vi "AI-Freq1.vi"(7 "DAQConfigRef":T1, 8 "error in":errorcluster, 10 "Mode":string, 11 "CH":string) -> (0 "error out":errorcluster, 3 "波形图":waveform(dbl)(graph))   [LabVIEW 2013]
uses:
  Controls/DAQConfigRef.ctl
  Controls/DAQConfig.ctl
  <vilib>/DAQmx/read.llb/DAQmx Read (Analog Wfm 1Chan NSamp).vi
  <vilib>/DAQmx/create/channels.llb/DAQmx Create Channel (AI-Voltage-Basic).vi
  <vilib>/DAQmx/configure/timing.llb/DAQmx Timing (Sample Clock).vi
  <vilib>/DAQmx/miscellaneous.llb/DAQmx Fill In Error Info.vi
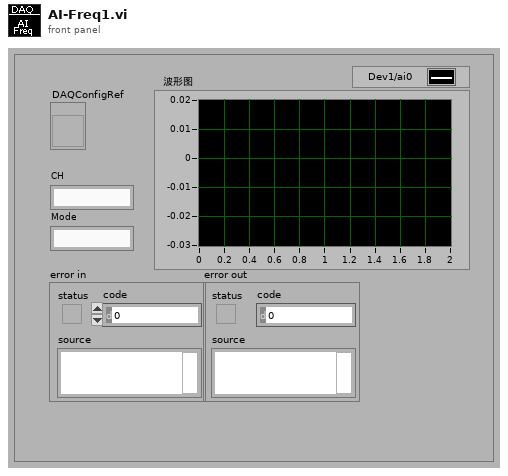
[diagram p1: front panel]
types:
  T1 = typedef "DAQConfigRef.ctl" = refnum<vi>
  T2 = typedef "DAQConfig.ctl" = cluster{"DIO":string[][], "AO":string[][], "AI":string[][]}
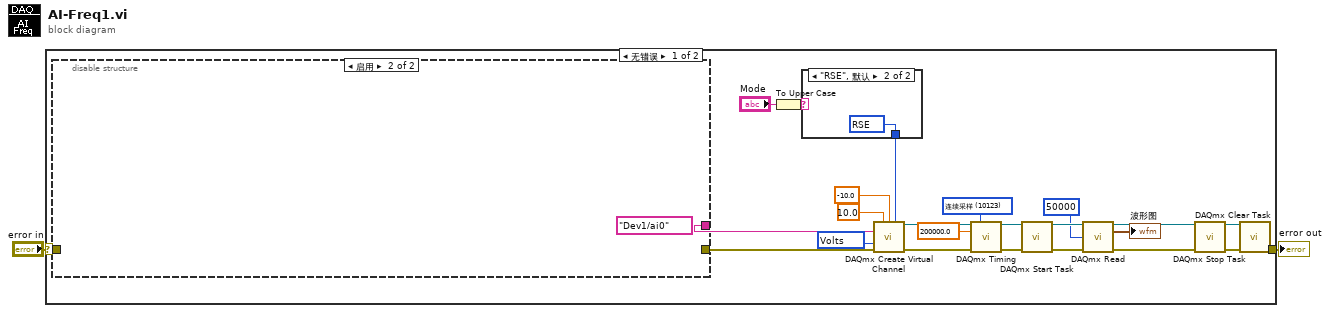
[diagram p0: block diagram]
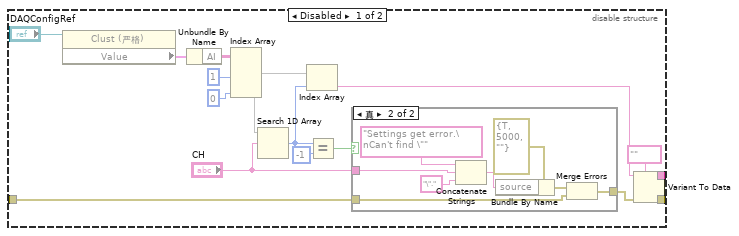
[diagram p2: hidden frame]
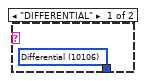
[diagram p4: hidden frame]
diagram:
  n1 = case shown="无错误" "error in" {
    selector: "error in" -> [w15 w56]
    tunnel: [w26 w56] -> w2
    frame No Error {
      w11 = 10123 items=["有限采样"=10178, "连续采样"=10123, "硬件定时单点"=12522] ("sample mode")
      w21 = 10348 items=["Volts"=10348, "From Custom Scale"=10065] ("units")
      n2 = disable-structure shown="启用" {
        disable-tunnel: [w31 tag "Dev1/ai0" ("lines")] -> w17
        disable-tunnel: [w30 _] -> w16
        disable-tunnel: w15 -> [w28 _]
        frame Disabled {
          n3 = property class="Clust (严格)"(reference="DAQConfigRef") -> ("Value"=w38:T2)  [unwired: 1 in, 2 out]
          n4 = Unbundle By Name(w38) -> ("AI"=w43:string[][])
          n5 = Index Array(array=w43, index (col) #1=1 ("索引 (行)"), index (col) #2=0 ("索引 (列)")) -> (element #1=w37:string[], element #2=w36:string[])  [unwired: 2 in]
          n6 = Search 1D Array(1D array=w36, element="CH") -> (index of element=w40:i32)  [unwired: 1 in]
          n7 = Index Array(array=w37, index=w40) -> (element=w27:string)
          n8 = Equal?(x=w40, y=-1) -> (x = y?=w34:bool)
          n9 = case shown="真" w34 {
            tunnel: w28 -> [w44 w47]
            tunnel: [w44 w46] -> w29
            tunnel: "CH" -> [_ w45]
            frame False {
            }
            frame True {
              n10 = Concatenate Strings("Settings get error.\nCan't find \"" ("message"), w45, "\"." ("string")) -> (w51:string)
              n11 = Bundle By Name(cluster=errorcluster {"status"=TRUE, "code"=5000, "source"=""} ("error in 1 (no error)"), "source"=w51) -> (w50:errorcluster)
              n12 = Merge Errors(w50, w47) -> (w46:errorcluster)
            }
          }
          n13 = Variant To Data(error in=w29, type=tag "" ("lines"), Variant=w27) -> (data=w31:tag, error out=w30:errorcluster)
        }
        frame Enabled {
        }
      }
      n14 = To Upper Case(1:"Mode") -> (0:w13:string)
      n15 = case shown="\"RSE\", 默认" w13 {
        tunnel: [w54 w55] -> w12
        frame "DIFFERENTIAL" {
          w54 = 10106 items=["default"=-1, "RSE"=10083, "NRSE"=10078, "Differential"=10106, "Pseudodifferential"=12529] ("input terminal configuration")
        }
        frame "RSE", Default {
          w55 = 10083 items=["default"=-1, "RSE"=10083, "NRSE"=10078, "Differential"=10106, "Pseudodifferential"=12529] ("input terminal configuration")
        }
      }
      n16 = call-poly <vilib>:"DAQmx Create Virtual Channel.vi"("maximum value"=10.0, "minimum value"=-10.0, "input terminal configuration"=w12, "physical channels"=w17, "units"=w21, "error in"=w16) -> ("task out"=w9:refnum<k21>, "error out"=w7:errorcluster)  [unwired: 8 in]
      n17 = call-poly <vilib>:"DAQmx Timing.vi"("task/channels in"=w9, "sample mode"=w11, "rate"=200000.0, "error in"=w7) -> ("task out"=w8:refnum<k21>, "error out"=w6:errorcluster)  [unwired: 3 in, 7 out]
      n18 = call <vilib>:"DAQmx Start Task.vi"("task/channels in"=w8, "error in"=w6) -> ("task out"=w25:refnum<k21>, "error out"=w24:errorcluster)  [unwired: 12 in]
      n19 = call-poly <vilib>:"DAQmx Read.vi"("task/channels in"=w25, "number of samples per channel"=50000, "error in"=w24) -> ("task out"=w20:refnum<k21>, "data"=→"波形图":waveform(dbl), "error out"=w4:errorcluster)  [unwired: 10 in]
      n20 = call <vilib>:"DAQmx Stop Task.vi"("task/channels in"=w20, "error in"=w4) -> ("task out"=w23:refnum<k21>, "error out"=w22:errorcluster)  [unwired: 12 in]
      n21 = call <vilib>:"DAQmx Clear Task.vi"("task in"=w23, "error in"=w22) -> ("error out"=w26:errorcluster)  [unwired: 13 in]
    }
    frame Error {
    }
  }
  "error out" <- w2
